vi "Ini_SetOutput.vi"(8 "error in (no error)":errorcluster, 11 "DMC1000B in":refnum<class "DMC1000B.lvclass">) -> (0 "error out":errorcluster, 3 "DMC1000B out":refnum<class "DMC1000B.lvclass">)   [LabVIEW 2019, in "DMC1000B.lvclass"]
uses:
  DMC1000B.lvclass
  IOCard.lvclass
  LLB/DMC1000B/Dmc1000/Dmc1000.lvlib
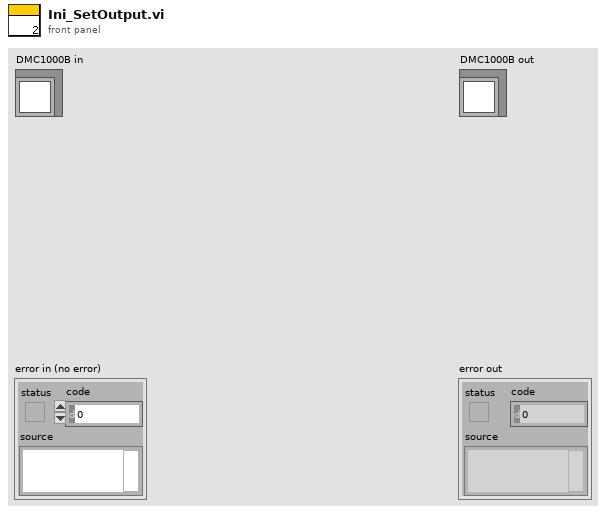
[diagram p1: front panel]
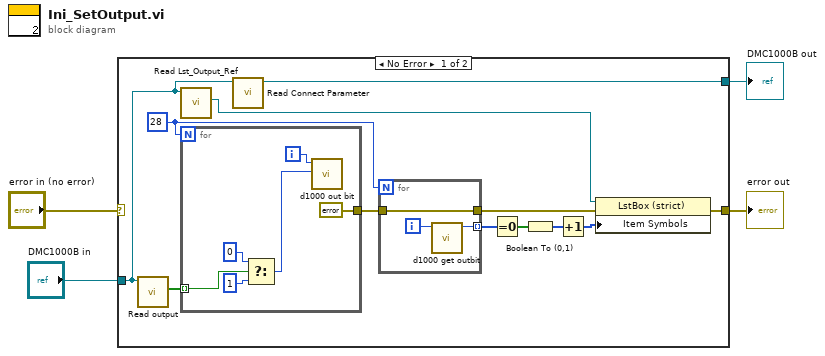
[diagram p0: block diagram]
diagram:
  n1 = case shown="No Error" "error in (no error)" {
    selector: "error in (no error)" -> [_ w27]
    tunnel: "DMC1000B in" -> [w6 w26]
    tunnel: [w14 w26] -> w2
    tunnel: [w13 w27] -> w1
    frame No Error {
      w10 = 28
      n2 = call-dynamic "Read output.vi"("IOCard in"=w6) -> ("output"=w5:bool[])  [unwired: 8 in, 2 out]
      n3 = call-dynamic "Read Lst_Output_Ref.vi"("IOCard in"=w6) -> ("Lst_Output_Ref"=w15:refnum<vi>)  [unwired: 8 in, 2 out]
      n4 = for {
        N: w10 -> [_]
        tunnel: [errorcluster {"status"=FALSE, "code"=0, "source"=""} ("error constant")] -> w12
        tunnel: w5 -> [w22] mode=indexing
        i -> [w25]
        n5 = Select(t=0, s=w22, f=1) -> (s? t:f=w23:i32)
        n6 = call "d1000 out bit.vi"("BitData"=w23, "BitNo"=w25) -> ()  [unwired: 9 in, 1 out]
      }
      n7 = call "Read Connect Parameter.vi"("IOCard in"=w6) -> ("IOCard out"=w14:refnum<class "DMC1000B.lvclass">)  [unwired: 8 in, 2 out]
      n8 = for {
        N: w10 -> [_]
        tunnel: [w19] -> w11
        tunnel: w12 -> [w19]
        tunnel: [w17] -> w8 mode=indexing
        i -> [w18]
        n9 = call "d1000 get outbit.vi"("BitNo"=w18) -> ("function return"=w17:u32)  [unwired: 10 in]
      }
      n10 = Equal To 0?(x=w8) -> (x = 0?=w7:bool[])
      n11 = Boolean To (0,1)(Boolean=w7) -> (0, 1=w16:i16[])
      n12 = Increment(x=w16) -> (x+1=w9:i16[])
      n13 = property class="LstBox (strict)"(reference=w15, error in=w11, "Item Symbols"=w9) -> (error out=w13:errorcluster)  [unwired: 1 out]
    }
    frame Error {
    }
  }
  "error out" <- w1
  "DMC1000B out" <- w2
